vi "BB_Check_Camera_IP_Change.vi"(11 "Incoming IP":string) -> (2 "Operation":enum16{"Read", "Reopen", "Close"}(ring))   [LabVIEW 2012]
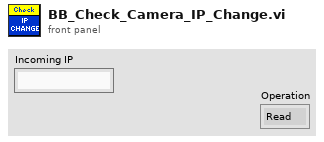
[diagram p1: front panel]
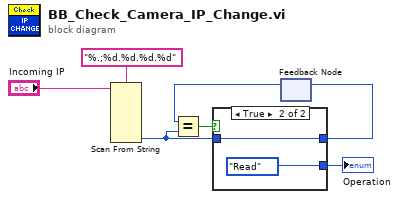
[diagram p0: block diagram]
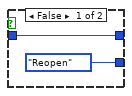
[diagram p2: hidden frame]
diagram:
  n1 = Scan From String(format string="%.;%d.%d.%d.%d", input string="Incoming IP") -> (output 4=w5:i32)  [unwired: 2 in, 10 out]
  n2 = feedback #1() -> (w1:i32)  [unwired: 1 in]
  n3 = Equal?(x=w1, y=w5) -> (x = y?=w3:bool)
  n4 = case shown="True" w3 {
    tunnel: w5 -> [w8 w11]
    tunnel: [w8 w11] -> w2
    tunnel: [enum16{"Read", "Reopen", "Close"}."Reopen" ("Operation") enum16{"Read", "Reopen", "Close"}."Read" ("Operation")] -> w4
    frame False {
    }
    frame True {
    }
  }
  "Operation" <- w4
  n5 = feedback-in #1(w2) -> ()
